vi "Read.vi"(8 "error in (no error)":errorcluster, 11 "HTTP Command Config in":refnum<class "HTTP Command Config.lvclass">) -> (0 "error out":errorcluster, 1 "Payload":string, 2 "URL":string, 3 "HTTP Command Config out":refnum<class "HTTP Command Config.lvclass">, 4 "Timeout":i32)   [LabVIEW 2023, in "VolatusSeqConfig.lvlib" / "HTTP Command Config.lvclass"]
uses:
  HTTP Command Config.lvclass
  HTTP Command Config.lvclass/HTTP Command Config.ctl
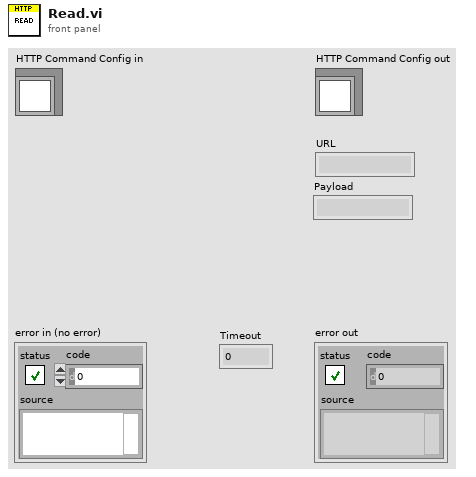
[diagram p1: front panel]
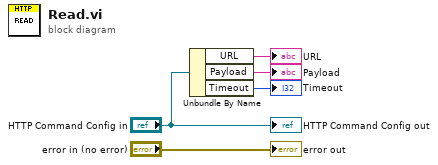
[diagram p0: block diagram]
diagram:
  n1 = Unbundle By Name("HTTP Command Config in") -> ("URL"=→"URL":string, "Payload"=→"Payload":string, "Timeout"=→"Timeout":i32)
  "error out" <- "error in (no error)"
  "HTTP Command Config out" <- "HTTP Command Config in"
